vi "Initialize Generate.vi"(8 "error in (no error)":errorcluster, 10 "PCL (usec)":u32, 11 "OnCompile Variables":T1={"Name"="", "XNET Settings"={"Database"="", "Cluster"="", "Port"="", "Baud rate [Bd]"=500000, "Termination"=1, "CAN I/O Mode"=0, "FD Baud rate [Bd]"=500000, "Priority"=100, "Use Legacy"=FALSE, "FD ISO Mode"=0}, "Frames"=[], "986x Support"={"Enable"=FALSE, "RIO Device"="", "Bitfile"=path ""}, "Incoming Frames"=[]} {"Incoming Frames"."Protection Configurations"."CRC Channels"."Data Type" items=["Signed", "Unsigned", "IEEE Float"]; "XNET Settings"."FD ISO Mode" items=["ISO", "Non ISO", "ISO Legacy"]; "XNET Settings"."CAN I/O Mode" items=["CAN 2.0", "CAN FD", "CAN FD+BRS"]; "XNET Settings"."Termination" items=["Off", "On"]; "Frames"."Protection Configurations"."CRC Channels"."Data Type" items=["Signed", "Unsigned", "IEEE Float"]}) -> (0 "error out":errorcluster, 2 "RT Configuration":T11={"Name"="", "Priority"=100, "XNET Settings"={"Database"="", "Cluster"="", "Port"="", "Baud rate [Bd]"=0, "Termination"=0, "CAN I/O Mode"=0, "FD Baud rate [Bd]"=500000, "Priority"=100, "Use Legacy"=FALSE, "FD ISO Mode"=0}, "FPGA Session"=0, "Outgoing CAN Session"="", "Outgoing Frame Count"=0, "Outgoing Frames"=[], "Incoming CAN Session"="", "Incoming Frame Count"=0, "Incoming Frames"=[], "Incoming Values"={"Signal Values"=[], "Signal Invalid Values"=[], "ProtCtr Sig Values"=[], "Timestamps"=[], "Time Differences"=[], "IDs"=[]}} {"Incoming Frames"."Protection Configurations"."CRC Channels"."Data Type" items=["Signed", "Unsigned", "IEEE Float"]; "XNET Settings"."FD ISO Mode" items=["ISO", "Non ISO", "ISO Legacy"]; "XNET Settings"."CAN I/O Mode" items=["CAN 2.0", "CAN FD", "CAN FD+BRS"]; "XNET Settings"."Termination" items=["Off", "On"]; "Outgoing Frames"."Protection Configurations"."CRC Channels"."Data Type" items=["Signed", "Unsigned", "IEEE Float"]}, 3 "OnCompile Variables out":T1={"Name"="", "XNET Settings"={"Database"="", "Cluster"="", "Port"="", "Baud rate [Bd]"=500000, "Termination"=1, "CAN I/O Mode"=0, "FD Baud rate [Bd]"=500000, "Priority"=100, "Use Legacy"=FALSE, "FD ISO Mode"=0}, "Frames"=[], "986x Support"={"Enable"=FALSE, "RIO Device"="", "Bitfile"=path ""}, "Incoming Frames"=[]} {"Incoming Frames"."Protection Configurations"."CRC Channels"."Data Type" items=["Signed", "Unsigned", "IEEE Float"]; "XNET Settings"."FD ISO Mode" items=["ISO", "Non ISO", "ISO Legacy"]; "XNET Settings"."CAN I/O Mode" items=["CAN 2.0", "CAN FD", "CAN FD+BRS"]; "XNET Settings"."Termination" items=["Off", "On"]; "Frames"."Protection Configurations"."CRC Channels"."Data Type" items=["Signed", "Unsigned", "IEEE Float"]})   [LabVIEW 2019, in "Ghost Bus Addon Engine.lvlib"]
uses:
  Ghost Bus Addon Engine.lvlib
  Addon Shared/Types/Exported.OnCompile.ctl
  Addon Shared/Types/XNET Settings.ctl
  SubModules/Frame-Protection-Support/Source/Shared/Types/Exported Frame Settings.ctl
  SubModules/Frame-Protection-Support/Source/Shared/Types/Exported Frame Type.ctl
  SubModules/Frame-Protection-Support/Source/Shared/Types/Exported Protection Settings.ctl
  SubModules/Frame-Protection-Support/Source/Shared/Types/Protection Type.ctl
  SubModules/Frame-Protection-Support/Source/Shared/Types/XNET Signal Configuration.ctl
  SubModules/Frame-Protection-Support/Source/Shared/Types/Exported Counter Settings.ctl
  SubModules/Frame-Protection-Support/Source/Shared/Types/Exported Event Trigger Type.ctl
  Addon Shared/Types/986x.ctl
  Types/RT Async Engine Settings.ctl
  SubModules/Frame-Protection-Support/Source/Engine/Types/RT Frame Settings.ctl
  SubModules/Frame-Protection-Support/Source/Engine/Types/RT Protection Configuration.ctl
  SubModules/Frame-Protection-Support/Source/Engine/Types/RT Frame Incoming Values.ctl
  Bitfile.Download.vi
  <vilib>/Utility/libraryn.llb/Check if File or Folder Exists.vi
  <vilib>/Utility/error.llb/Error Cluster From Error Code.vi
  <vilib>/rvi/Utilities/XML/nirviXML_GetValue.vi
  <vilib>/rvi/Utilities/XML/nirviXML_GetValue_String.vi
  <vilib>/xnet/xnet.llb/XNET Create Session (Frame Output Stream).vi
  <vilib>/xnet/xnet.llb/XNET Create Session (Conversion).vi
  SubModules/Frame-Protection-Support/Source/Shared/Protection and Counter Support Shared.lvlib
  SubModules/Frame-Protection-Support/Source/Engine/Protection and Counter Support Engine.lvlib
  <resource>/objmgr/xnet.rc
  Addon Shared/Ghost Bus Addon Shared.lvlib
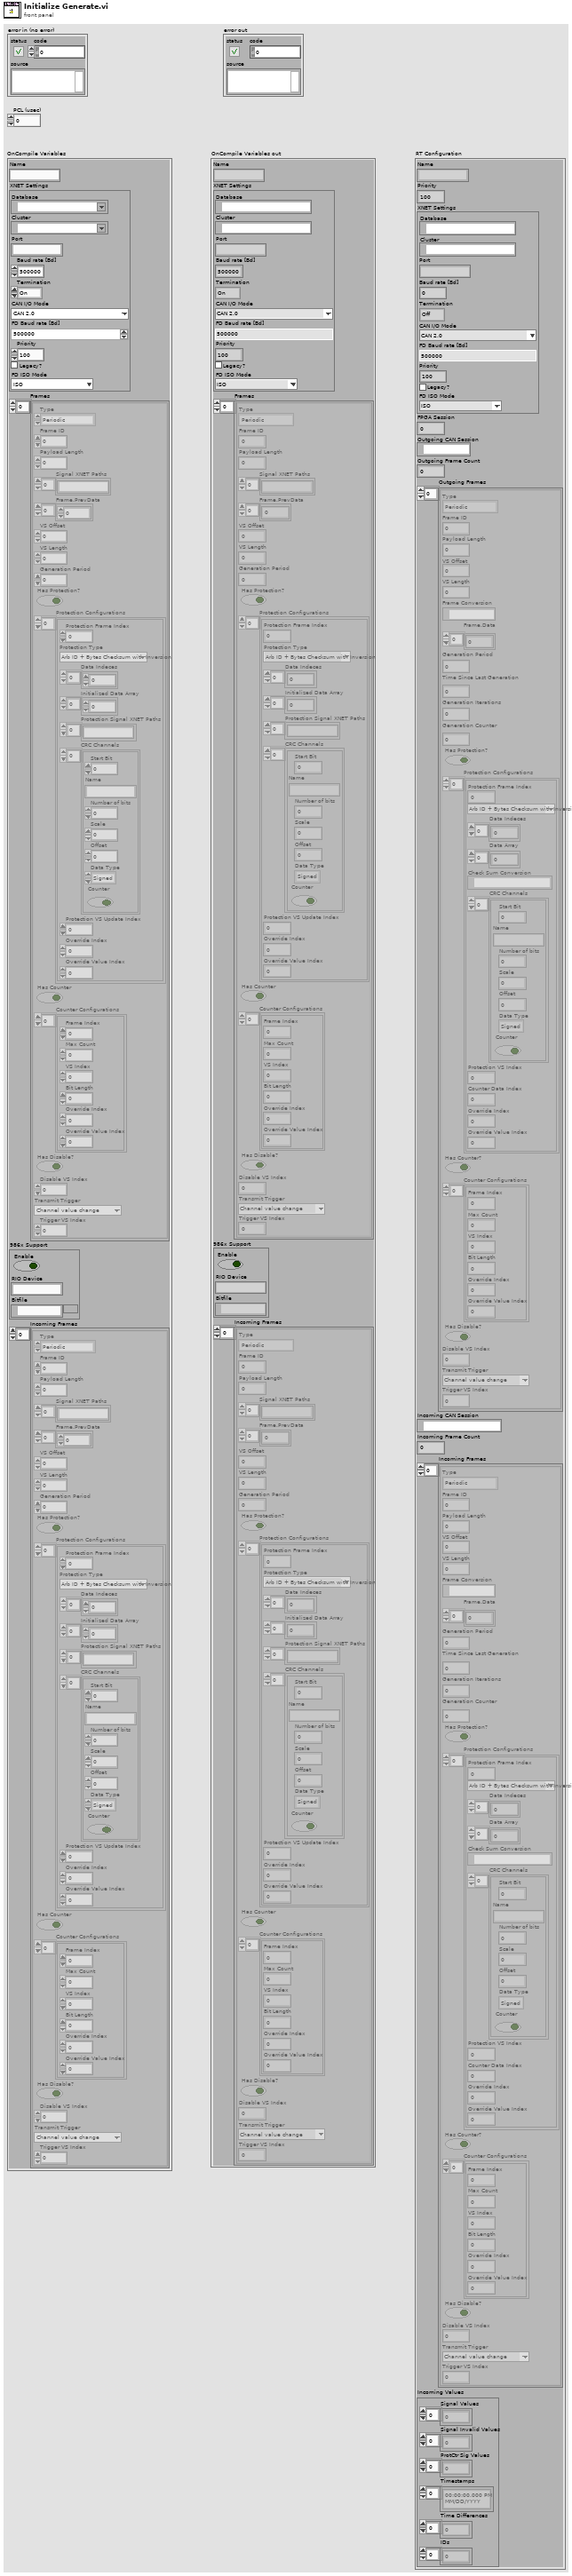
[diagram p1: front panel]
types:
  T1 = typedef "Ghost Bus Addon Shared.lvlib/Exported.OnCompile.ctl" = cluster{"Name":string, "XNET Settings":T2, "Frames":T3[], "986x Support":T10, "Incoming Frames":T3[]}
  T2 = typedef "Ghost Bus Addon Shared.lvlib/XNET Settings.ctl" = cluster{"Database":refnum<k21>, "Cluster":refnum<k21>, "Port":string, "Baud rate [Bd]":u64, "Termination":u32, "CAN I/O Mode":u32, "FD Baud rate [Bd]":u64, "Priority":i32, "Use Legacy":bool, "FD ISO Mode":u32}
  T3 = typedef "Protection and Counter Support Shared.lvlib/Exported Frame Settings.ctl" = cluster{"Type":T4, "Frame ID":u32, "Payload Length":u32, "Signal XNET Paths":string[], "Frame.PrevData":dbl[], "VS Offset":i32, "VS Length":i32, "Generation Period":u32, "Has Protection?":bool, "Protection Configurations":T5[], "Has Counter":bool, "Counter Configurations":T8[], "Has Disable?":bool, "Disable VS Index":i32, "Transmit Trigger":T9, "Trigger VS Index":i32}
  T4 = typedef "Protection and Counter Support Shared.lvlib/Exported Frame Type.ctl" = enum16{"Periodic", "Event", "Periodic/Event"}
  T5 = typedef "Protection and Counter Support Shared.lvlib/Exported Protection Settings.ctl" = cluster{"Protection Frame Index":i32, "Protection Type":T6, "Data Indeces":i32[], "Initialized Data Array":dbl[], "Protection Signal XNET Paths":string[], "CRC Channels":T7[], "Protection VS Update Index":i32, "Override Index":i32, "Override Value Index":i32}
  T6 = typedef "Protection and Counter Support Shared.lvlib/Protection Type.ctl" = enum16{"Arb ID + Bytes Checksum with Inversion", "Arb ID + Bytes CRC with Inversion", "Reversed Raw Signal Checksum with Inversion", "Concatenated Two's Compliment"}
  T7 = typedef "Protection and Counter Support Shared.lvlib/XNET Signal Configuration.ctl" = cluster{"Start Bit":i32, "Name":string, "Number of bits":i32, "Scale":dbl, "Offset":dbl, "Data Type":u32, "Counter":bool}
  T8 = typedef "Protection and Counter Support Shared.lvlib/Exported Counter Settings.ctl" = cluster{"Frame Index":i32, "Max Count":dbl, "VS Index":i32, "Bit Length":i64, "Override Index":i32, "Override Value Index":i32}
  T9 = typedef "Protection and Counter Support Shared.lvlib/Exported Event Trigger Type.ctl" = enum16{"Channel value change", "Trigger channel (not zero)", "Channel value change or trigger channel (not zero)", "Trigger channel (any value change)", "Channel value change or trigger channel (any value change)"}
  T10 = typedef "Ghost Bus Addon Shared.lvlib/986x.ctl" = cluster{"Enable":bool, "RIO Device":string, "Bitfile":path}
  T11 = typedef "Ghost Bus Addon Engine.lvlib/RT Async Engine Settings.ctl" = cluster{"Name":string, "Priority":i32, "XNET Settings":T2, "FPGA Session":u32, "Outgoing CAN Session":refnum<k21>, "Outgoing Frame Count":i32, "Outgoing Frames":T12[], "Incoming CAN Session":refnum<k21>, "Incoming Frame Count":i32, "Incoming Frames":T12[], "Incoming Values":T14}
  T12 = typedef "Protection and Counter Support Engine.lvlib/RT Frame Settings.ctl" = cluster{"Type":T4, "Frame ID":u32, "Payload Length":u32, "VS Offset":i32, "VS Length":i32, "Frame Conversion":refnum<k21>, "Frame.Data":dbl[], "Generation Period":u32, "Time Since Last Generation":u32, "Generation Iterations":u32, "Generation Counter":u32, "Has Protection?":bool, "Protection Configurations":T13[], "Has Counter?":bool, "Counter Configurations":T8[], "Has Disable?":bool, "Disable VS Index":i32, "Transmit Trigger":T9, "Trigger VS Index":i32}
  T13 = typedef "Protection and Counter Support Engine.lvlib/RT Protection Configuration.ctl" = cluster{"Protection Frame Index":i32, "Protection Type":T6, "Data Indeces":i32[], "Data Array":dbl[], "Check Sum Conversion":refnum<k21>, "CRC Channels":T7[], "Protection VS Index":i32, "Counter Data Index":i32, "Override Index":i32, "Override Value Index":i32}
  T14 = typedef "Protection and Counter Support Engine.lvlib/RT Frame Incoming Values.ctl" = cluster{"Signal Values":dbl[], "Signal Invalid Values":dbl[], "ProtCtr Sig Values":dbl[], "Timestamps":timestamp[], "Time Differences":dbl[], "IDs":u32[]}
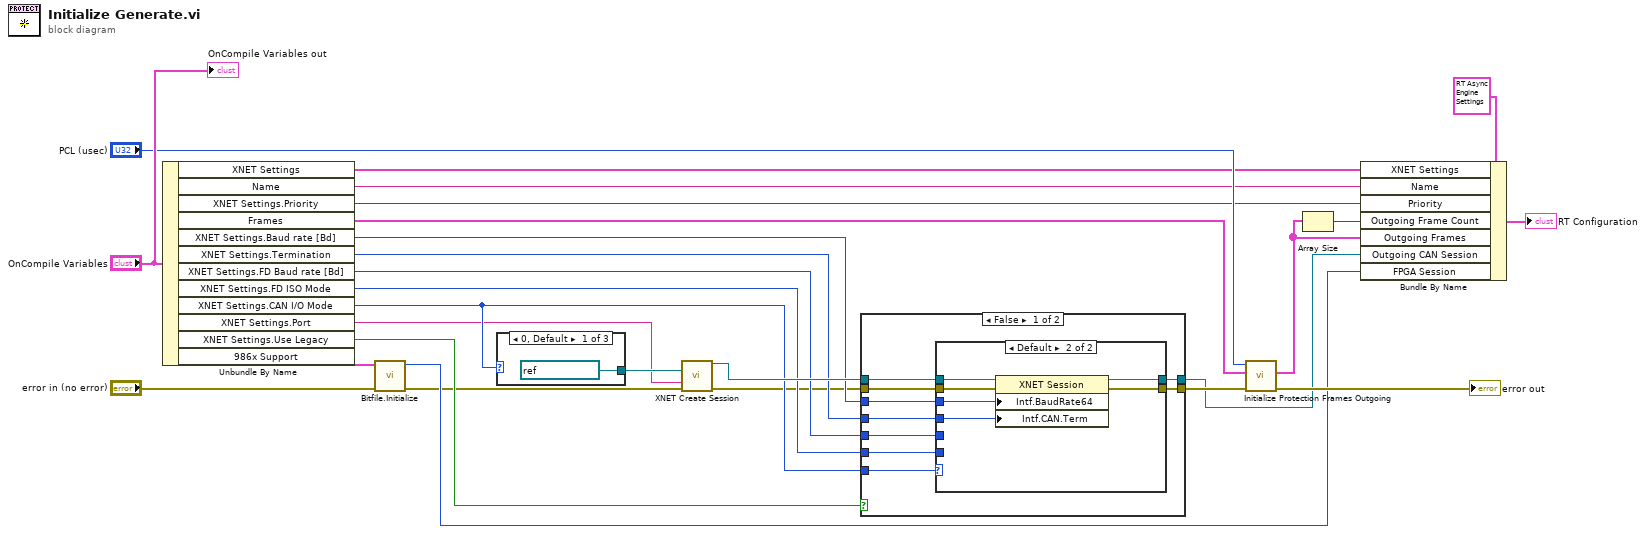
[diagram p0: block diagram]
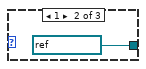
[diagram p2: hidden frame]
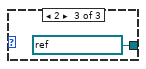
[diagram p3: hidden frame]
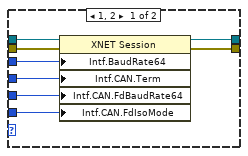
[diagram p4: hidden frame]
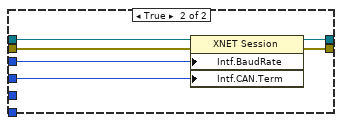
[diagram p5: hidden frame]
diagram:
  n1 = Unbundle By Name("OnCompile Variables") -> ("XNET Settings"=w8:T2, "Name"=w9:string, "XNET Settings.Priority"=w15:i32, "Frames"=w26:T3[], "XNET Settings.Baud rate [Bd]"=w18:u64, "XNET Settings.Termination"=w19:u32, "XNET Settings.FD Baud rate [Bd]"=w20:u64, "XNET Settings.FD ISO Mode"=w6:u32, "XNET Settings.CAN I/O Mode"=w5:u32, "XNET Settings.Port"=w1:string, "XNET Settings.Use Legacy"=w14:bool, "986x Support"=w13:T10)
  n2 = call "Bitfile.Initialize.vi"("error in (no error)"="error in (no error)", "FPGA Bitfile Settings"=w13) -> ("error out"=w3:errorcluster, "FPGA Session"=w12:u32)  [unwired: 8 in]
  n3 = case shown="0, Default" w5 {
    tunnel: [refnum<k21> ":memory:" ("cluster (:memory:)") refnum<k21> ":can_fd:" ("cluster (:memory:)") refnum<k21> ":can_fd_brs:" ("cluster (:memory:)")] -> w7
    frame 0, Default {
    }
    frame 1 {
    }
    frame 2 {
    }
  }
  n4 = call-poly <vilib>:"XNET Create Session.vi"("cluster (:memory:)"=w7, "interface"=w1, "error in (no error)"=w3) -> ("session out"=w22:refnum<k21>, "error out"=w2:errorcluster)  [unwired: 11 in]
  n5 = case shown="False" w14 {
    tunnel: w2 -> [w39 w59]
    tunnel: w22 -> [w38 w58]
    tunnel: [w37 w57] -> w21
    tunnel: w20 -> [w36 _]
    tunnel: w5 -> [w32 _]
    tunnel: w19 -> [w35 w54]
    tunnel: w18 -> [w34 w55]
    tunnel: [w33 w56] -> w10
    tunnel: w6 -> [w31 _]
    frame False {
      n6 = case shown="Default" w32 {
        tunnel: w39 -> [w47 w53]
        tunnel: w38 -> [w46 w52]
        tunnel: [w45 w51] -> w37
        tunnel: w36 -> [w44 _]
        tunnel: w35 -> [w43 w50]
        tunnel: w34 -> [w42 w49]
        tunnel: [w41 w48] -> w33
        tunnel: w31 -> [w40 _]
        frame 1, 2 {
          n7 = property class="XNET Session"(reference=w46, error in=w47, "Intf.BaudRate64"=w42, "Intf.CAN.Term"=w43, "Intf.CAN.FdBaudRate64"=w44, "Intf.CAN.FdIsoMode"=w40) -> (reference out=w41:refnum<k21>, error out=w45:errorcluster)
        }
        frame Default {
          n8 = property class="XNET Session"(reference=w52, error in=w53, "Intf.BaudRate64"=w49, "Intf.CAN.Term"=w50) -> (reference out=w48:refnum<k21>, error out=w51:errorcluster)
        }
      }
    }
    frame True {
      n9 = property class="XNET Session"(reference=w58, error in=w59, "Intf.BaudRate"=w55, "Intf.CAN.Term"=w54) -> (reference out=w56:refnum<k21>, error out=w57:errorcluster)
    }
  }
  n10 = call "Initialize Protection Frames Outgoing.vi"("error in (no error)"=w21, "Frames"=w26, "PCL (usec)"="PCL (usec)") -> ("error out"=→"error out":errorcluster, "RT Frames"=w11:T12[])  [unwired: 7 in]
  n11 = Array Size(array=w11) -> (size(s)=w16:i32)
  n12 = Bundle By Name(cluster=T11 {"Name"="", "Priority"=100, "XNET Settings"={"Database"="", "Cluster"="", "Port"="", "Baud rate [Bd]"=0, "Termination"=0, "CAN I/O Mode"=0, "FD Baud rate [Bd]"=500000, "Priority"=100, "Use Legacy"=FALSE, "FD ISO Mode"=0}, "FPGA Session"=0, "Outgoing CAN Session"="", "Outgoing Frame Count"=0, "Outgoing Frames"=[], "Incoming CAN Session"="", "Incoming Frame Count"=0, "Incoming Frames"=[], "Incoming Values"={"Signal Values"=[], "Signal Invalid Values"=[], "ProtCtr Sig Values"=[], "Timestamps"=[], "Time Differences"=[], "IDs"=[]}} ("RT Configuration"), "XNET Settings"=w8, "Name"=w9, "Priority"=w15, "Outgoing Frame Count"=w16, "Outgoing Frames"=w11, "Outgoing CAN Session"=w10, "FPGA Session"=w12) -> (→"RT Configuration":T11)
  "OnCompile Variables out" <- "OnCompile Variables"
